vi "Get Versions of All Controllers (uSMC).vi"(8 "error in":errorcluster, 10 "axis":i32, 11 "Visa array in":refnum<visa-resource-name>[](array[refnum])) -> (0 "error out":errorcluster, 1 "Versions":string, 3 "Visa array out":refnum<visa-resource-name>[](array[refnum]))   [LabVIEW 2010, in "SignalWriterMH110203USBStepperMotor.lvclass"]
uses:
  SignalWriterMH110203USBStepperMotor.lvclass
  class_data.vi
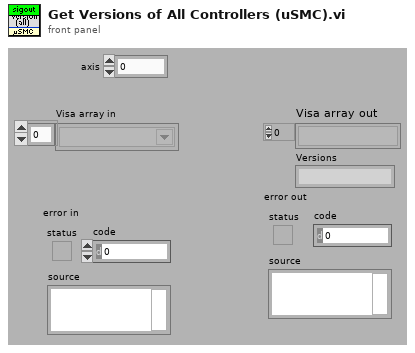
[diagram p1: front panel]
types:
  T1 = typedef "SignalWriterMH110203USBStepperMotor.lvclass/GoTo Control (uSMC).ctl" = cluster{"Step motor ID":string, "SMname":string, "Backlash":u16, "wait for input sygnal to start":bool, "use slow start/stop":bool, "units name":string, "Maximum speed":dbl, "speed":dbl, "step":u8, "point 1 ticks":i32, "point 2 ticks":i32, "point 1 units":dbl, "point 2 units":dbl, "Limit Switch standoff":dbl, "Zero Value":dbl, "Destination Position":dbl, "force backlash":bool, "power off when stop":bool, "POff delay":dbl, "positioner name":string, "R, Ohm":dbl, "I, mA":dbl, "Positioner's Type":u16, "Reset Direction":bool, "Manufacturer":string, "Model":string, "Scheme":string, "FirmwareVer":string}
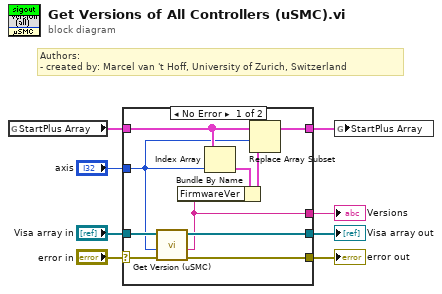
[diagram p0: block diagram]
diagram:
  # "Authors: \n- created by: Marcel van 't Hoff, University of Zurich, Switzerland"
  n1 = global read "class_data.vi" "StartPlus Array"() -> (w4:T1[])
  n2 = case shown="No Error" "error in" {
    selector: "error in" -> [w9 w21]
    tunnel: [w18 w20] -> w8
    tunnel: [w17 w21] -> w7
    tunnel: "Visa array in" -> [w16 w20]
    tunnel: [w14 _] -> w5
    tunnel: w4 -> [w13 w19]
    tunnel: [w11 w19] -> w3
    tunnel: "axis" -> [w10 _]
    frame No Error {
      n3 = call "Get Version (uSMC).vi"("error in (no error)"=w9, "Index"=w10, "Visa array in"=w16) -> ("error out"=w17:errorcluster, "Firmware Version"=w14:string, "Visa array out"=w18:refnum<visa-resource-name>[])  [unwired: 6 in]
      n4 = Index Array(array=w13, index=w10) -> (element=w15:T1)
      n5 = Bundle By Name(cluster=w15, "FirmwareVer"=w14) -> (w12:T1)
      n6 = Replace Array Subset(array=w13, new element=w12, index=w10) -> (w11:T1[])
    }
    frame Error {
    }
  }
  "Visa array out" <- w8
  "error out" <- w7
  "Versions" <- w5
  n7 = global write "class_data.vi" "StartPlus Array"(w3) -> ()
